vi "Start.vi"(0 "reference in":refnum<class "sim_MmW.lvclass">, 5 "TX bursts":refnum<class "mmWave data.lvclass">[](array[class]), 7 "sequence":string[](array[string]), 9 "RX acq duration":dbl=320000.0, 11 "error in (no error)":errorcluster) -> (4 "reference out":refnum<class "sim_MmW.lvclass">, 15 "error out":errorcluster)   [LabVIEW 2019, in "sim_MmW.lvclass"]
doc: "Starts insturment operation:"
uses:
  sim_MmW.lvclass
  C:/Barkhausen mmWave radar/Development/modules/mmw_instrument/src_LabVIEW/Host/SubVIs/mmWave instrument_class/mmWave instrument.lvclass
  mmWave data_class/mmWave data.lvclass
  mmWave instrument_class/Instrument state.ctl
  mmWave HW Control/HW custom error.ctl
  mmWave instrument_class/mmWave instrument.lvclass
  mmWave HW Control/mmWave HW Control.lvlib
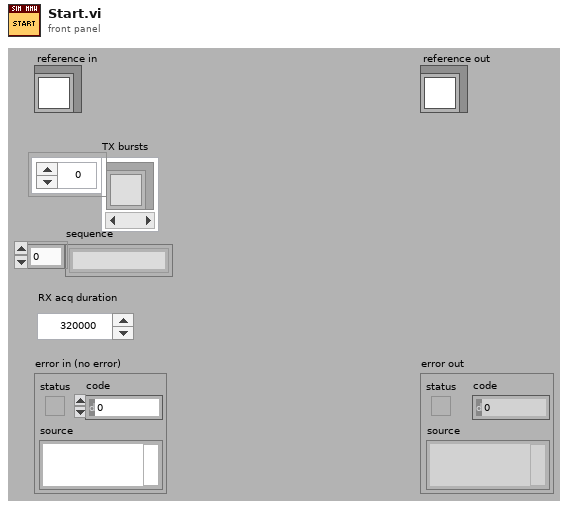
[diagram p1: front panel]
types:
  T1 = typedef "mmWave instrument.lvclass/Instrument state.ctl" = enum16{"Off", "Initialization", "Configuration", "Running", "Calibration"}
  T2 = typedef "mmWave instrument.lvclass/ObjectAttributes.ctl" = cluster{"mode":T3, "instr state":T1, "Max Fs":dbl, "Equalization coeff":cdb[], "LO sync en":bool, "Trig sync en":bool, "LO sources":T4, "LO Export":T5, "Fc.range":cluster{"min":dbl, "max":dbl}, "Sync mode":T6, "equalization en":bool, "sequence":string[]}
  T3 = typedef "mmWave instrument.lvclass/Instrument mode.ctl" = enum16{"RF", "IF", "BB"}
  T4 = typedef "mmWave HW Control.lvlib/LO sources.ctl" = cluster{"RX/LO1 src":string, "TX/LO1 src":string, "LO2 src":string}
  T5 = typedef "mmWave HW Control.lvlib/LO export.ctl" = cluster{"TX LO1 export":bool, "TX LO1 export level":dbl, "RX LO1 export":bool, "RX LO1 export level":dbl, "LO2 export":bool, "LO2 export level":dbl}
  T6 = typedef "mmWave instrument.lvclass/Sync mode.ctl" = enum16{"Slave", "Master"}
  T7 = typedef "sim_MmW.lvclass/ObjectAttributesRef.ctl" = refnum<data-value>
  T8 = typedef "sim_MmW.lvclass/ObjectAttributes.ctl" = cluster{"RF config":T9, "RX samples":i32, "Downloaded Bursts":map{string, refnum<class "mmWave data.lvclass">}, "TX Fs":dbl, "RX Fs":dbl, "burst sequence":string[], "Burst mode":T10}
  T9 = typedef "mmWave HW Control.lvlib/HW TXRX RF config cluster.ctl" = cluster{"TX.Frequency":dbl, "TX.Gain":dbl, "TX.mmWave adapter":string, "RX.Frequency":dbl, "RX.Gain":dbl, "RX.mmWave adapter":string}
  T10 = typedef "mmWave instrument.lvclass/BurstMode.ctl" = enum16{"burst", "continuous"}
  T11 = typedef "mmWave HW Control.lvlib/HW custom error.ctl" = u16
  T12 = typedef "Constants.ctl" = cluster{"data clock rate (Hz)":dbl, "sample rate (Hz)":dbl, "sample rate selector string":string, "default tx bitfile path":path, "default rx bitfile path":path, "default proc bitfile path":path}
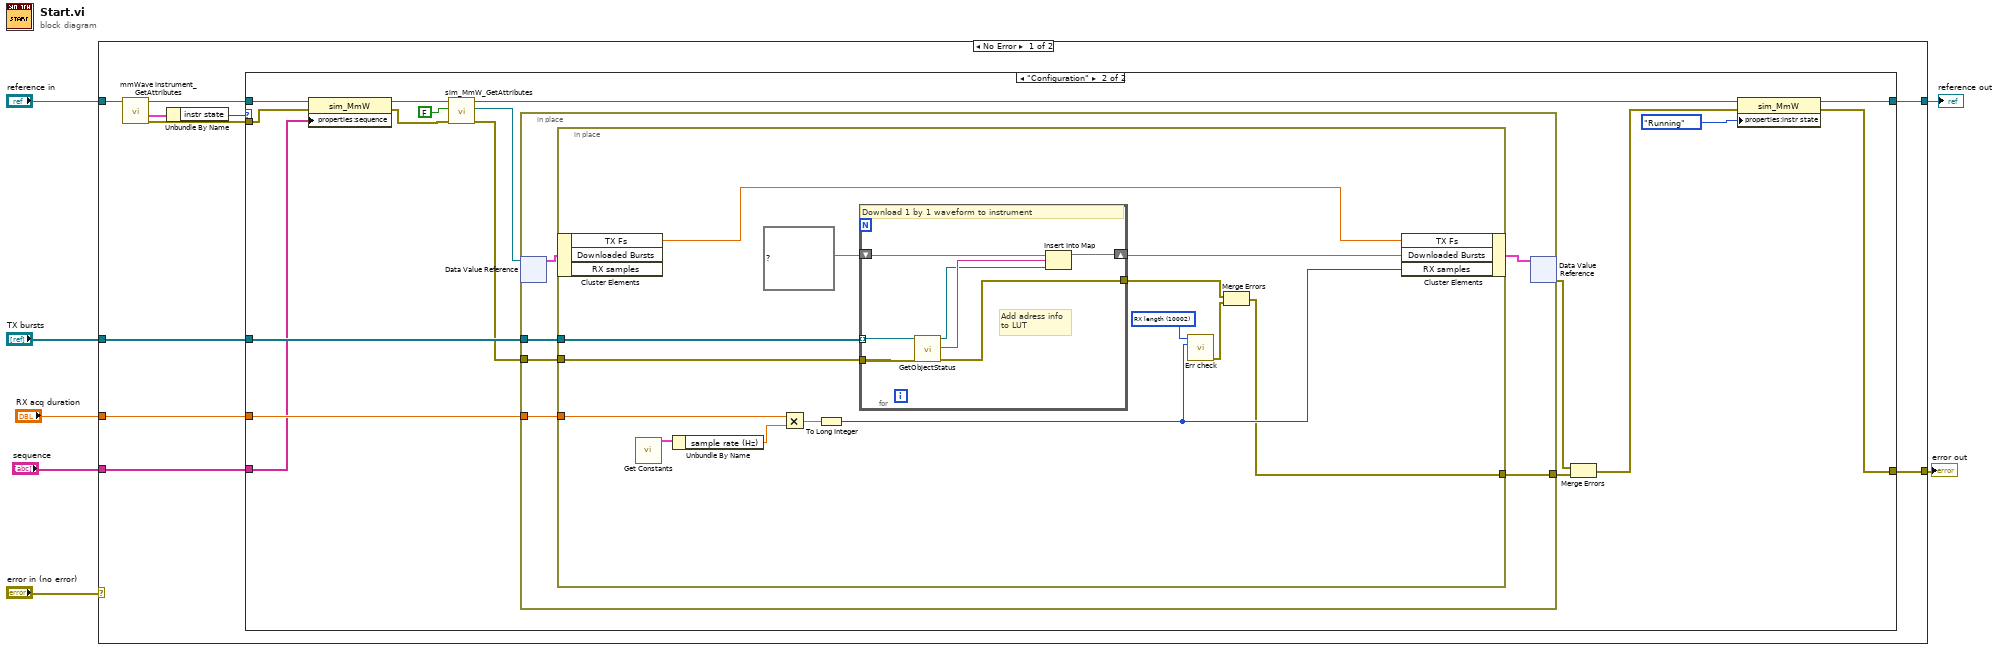
[diagram p0: block diagram]
diagram:
  n1 = case shown="No Error" "error in (no error)" {
    selector: "error in (no error)" -> [_ w64]
    tunnel: [w17 w64] -> w6
    tunnel: [w15 w63] -> w4
    tunnel: "reference in" -> [w16 w63]
    tunnel: "TX bursts" -> [w9 _]
    tunnel: "RX acq duration" -> [w10 _]
    tunnel: "sequence" -> [w8 _]
    frame No Error {
      n2 = call "mmWave instrument_GetAttributes.vi"("reference in"=w16) -> ("error out"=w11:errorcluster, "attributes"=w13:T2, "reference out"=w14:refnum<class "sim_MmW.lvclass">)  [unwired: 7 in, 1 out]
      n3 = Unbundle By Name(w13) -> ("instr state"=w12:T1)
      n4 = case shown="\"Configuration\"" w12 {
        tunnel: [_ w24] -> w17
        tunnel: [w18 w27] -> w15
        tunnel: w14 -> [w18 w23]
        tunnel: w9 -> [_ w31]
        tunnel: w11 -> [_ w20]
        tunnel: w10 -> [_ w30]
        tunnel: w8 -> [_ w21]
        frame "Off", Default {
        }
        frame "Configuration" {
          n5 = property class="sim_MmW"(reference=w23, error in=w20, "properties:sequence"=w21) -> (reference out=w22:refnum<class "sim_MmW.lvclass">, error out=w19:errorcluster)
          n6 = call "sim_MmW_GetAttributes.vi"("error in (no error)"=w19, "return data? (T)"=FALSE, "reference in"=w22) -> ("error out"=w29:errorcluster, "attributes ref"=w32:T7, "reference out"=w33:refnum<class "sim_MmW.lvclass">)  [unwired: 5 in, 1 out]
          n7 = in-place {
            in-place-border: w31 -> [w39]
            in-place-border: w30 -> [w38]
            in-place-border: w29 -> [w37]
            in-place-border: [w36] -> w28
            n8 = in-place-dvr #1(w32) -> (w40:T8)  [unwired: 1 out]
            n9 = in-place {
              in-place-border: w39 -> [w55]
              in-place-border: w38 -> [w48]
              in-place-border: w37 -> [w54]
              in-place-border: [w45] -> w36
              w52 = T11 10002 items=["TX list"=10000, "TX length"=10001, "RX length"=10002] ("HW custom err")
              n10 = in-place-cluster #2(w40) -> ("TX Fs"=w49:dbl)  [unwired: 2 out]
              n11 = call "Get Constants.vi"() -> ("constants"=w44:T12)  [unwired: 15 in]
              n12 = Unbundle By Name(w44) -> ("sample rate (Hz)"=w43:dbl)
              n13 = Multiply(x=w48, y=w43) -> (x*y=w50:dbl)
              n14 = To Long Integer(number=w50) -> (32bit integer=w47:i32)
              n15 = for {
                tunnel: w55 -> [w60] mode=indexing
                tunnel: w54 -> [w58]
                shift-right: [w62] -> w42
                shift-left: map{string, refnum<class "mmWave data.lvclass">} {} ("Downloaded Bursts") -> [w61]
                tunnel: [w57] -> w46
                # "Add adress info\nto LUT"
                # "Download 1 by 1 waveform to instrument"
                n16 = call-dynamic "GetObjectStatus.vi"("reference in"=w60, "error in (no error)"=w58) -> ("reference out"=w56:refnum<class "mmWave data.lvclass">, "object name"=w59:string, "error out"=w57:errorcluster)  [unwired: 6 in, 9 out]
                n17 = Insert Into Map(map in=w61, key=w59, value=w56) -> (map out=w62:map{string, refnum<class "mmWave data.lvclass">})  [unwired: 2 out]
              }
              n18 = call "Err check.vi"("Variant Control"=w47, "HW custom err"=w52) -> ("error out"=w51:errorcluster)  [unwired: 9 in]
              n19 = Merge Errors(w46, w51) -> (w45:errorcluster)
              n20 = in-place-cluster #2("TX Fs"=w49, "Downloaded Bursts"=w42, "RX samples"=w47) -> (w41:T8)
            }
            n21 = in-place-dvr #1(w41) -> (w35:errorcluster)  [unwired: 1 out]
          }
          n22 = Merge Errors(w35, w28) -> (w26:errorcluster)
          n23 = property class="sim_MmW"(reference=w33, error in=w26, "properties:instr state"=Instrument_state."Running" ("instr state")) -> (reference out=w27:refnum<class "sim_MmW.lvclass">, error out=w24:errorcluster)
        }
      }
    }
    frame Error {
    }
  }
  "error out" <- w6
  "reference out" <- w4
